vi "Automatic CE-CERT Inverter MODBUS TCP-IP Curtailment.vi"() -> ()   [LabVIEW 2018]
uses:
  <vilib>/Plasmionique/MB Master/MB_Master_TCP/MB_Master_TCP.lvclass
  C:/Program Files (x86)/National Instruments/LabVIEW 2018/vi.lib/Plasmionique/MB Master/MB_Master/MB_Master.lvclass
  <vilib>/Plasmionique/MB Master/MB Master.lvlib
panel:
  in  "Curtailment Percentage (28-100%)":u16
  out "3035 Register Value":u16
  out "Curtailment Mode Read Back (Step 11)":u16
  out "Power Factor Mode Read Back (Step 10)":u16
  out "Power Factor Operation Error (Step 9)(Can Read 0 or 10)":u16
  out "Power Factor Operation Error (Step 1)(Should Read 0)":u16
  in  "IP Address":string
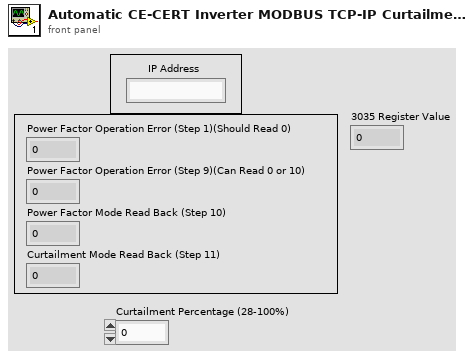
[diagram p1: front panel]
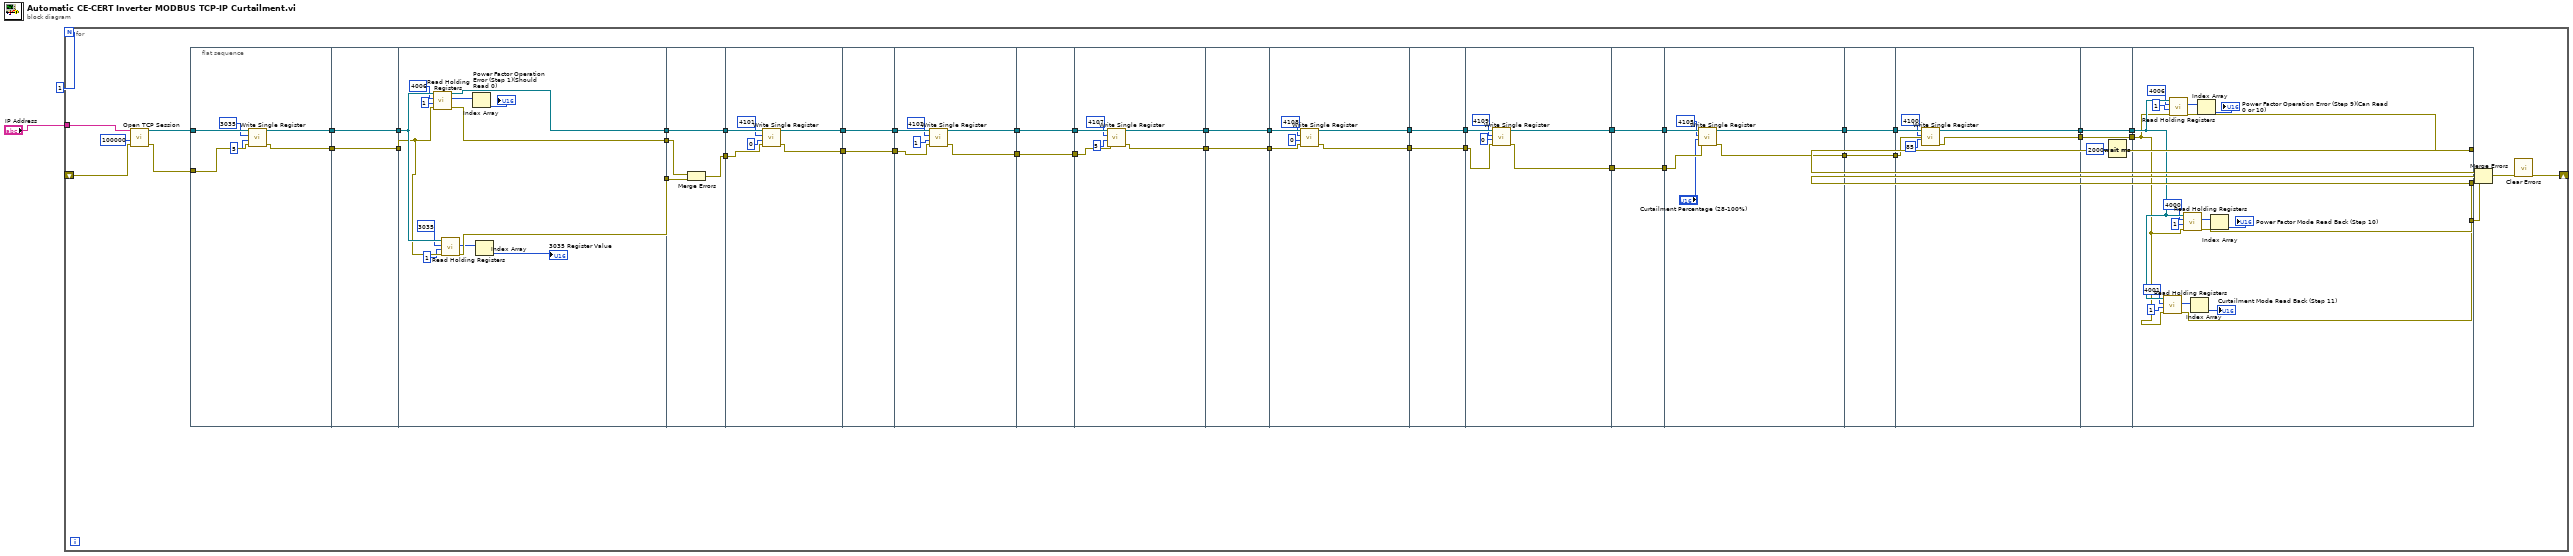
[diagram p0: block diagram]
diagram:
  n1 = for {
    N: 1 -> [_]
    tunnel: "IP Address" -> [w31]
    shift-right: [w5] -> _
    shift-left: _ -> [w4]
    n2 = call <vilib>:"Open TCP Session.vi"("error in (no error)"=w4, "Timeout (10000)"=100000, "IP Address"=w31) -> ("error out"=w29:errorcluster, "MB_TCP session"=w30:refnum<class "MB_Master_TCP.lvclass">)  [unwired: 7 in]
    n3 = flat-sequence {
      tunnel: w30 -> [w55]
      tunnel: [w54] -> w32
      tunnel: w29 -> [w53]
      tunnel: [w52] -> w27
      tunnel: [w57] -> w33
      tunnel: w32 -> [w57]
      tunnel: [w56] -> w28
      tunnel: w27 -> [w56]
      tunnel: [w70] -> w49
      tunnel: w33 -> [w69]
      tunnel: w28 -> [w68]
      tunnel: [w67] -> w25
      tunnel: [w66] -> w24
      tunnel: w49 -> [w74]
      tunnel: [w74] -> w48
      tunnel: [w71] -> w26
      tunnel: w25 -> [w73]
      tunnel: w24 -> [w72]
      tunnel: w48 -> [w80]
      tunnel: [w79] -> w47
      tunnel: w26 -> [w78]
      tunnel: [w77] -> w22
      tunnel: w47 -> [w82]
      tunnel: [w82] -> w46
      tunnel: [w81] -> w23
      tunnel: w22 -> [w81]
      tunnel: w46 -> [w88]
      tunnel: [w87] -> w45
      tunnel: w23 -> [w86]
      tunnel: [w85] -> w20
      tunnel: w45 -> [w90]
      tunnel: [w90] -> w44
      tunnel: [w89] -> w21
      tunnel: w20 -> [w89]
      tunnel: w44 -> [w96]
      tunnel: [w95] -> w43
      tunnel: w21 -> [w94]
      tunnel: [w93] -> w18
      tunnel: w43 -> [w98]
      tunnel: [w98] -> w42
      tunnel: [w97] -> w19
      tunnel: w18 -> [w97]
      tunnel: w42 -> [w104]
      tunnel: [w103] -> w41
      tunnel: w19 -> [w102]
      tunnel: [w101] -> w16
      tunnel: w41 -> [w106]
      tunnel: [w106] -> w40
      tunnel: [w105] -> w17
      tunnel: w16 -> [w105]
      tunnel: w40 -> [w112]
      tunnel: [w111] -> w39
      tunnel: w17 -> [w110]
      tunnel: [w109] -> w14
      tunnel: w39 -> [w114]
      tunnel: [w114] -> w38
      tunnel: [w113] -> w15
      tunnel: w14 -> [w113]
      tunnel: w38 -> [w120]
      tunnel: [w119] -> w37
      tunnel: w15 -> [w118]
      tunnel: [w117] -> w12
      tunnel: w37 -> [w122]
      tunnel: [w122] -> w36
      tunnel: [w121] -> w13
      tunnel: w12 -> [w121]
      tunnel: w36 -> [w128]
      tunnel: [w127] -> w35
      tunnel: w13 -> [w126]
      tunnel: [w125] -> w10
      tunnel: w35 -> [w131]
      tunnel: [w131] -> w34
      tunnel: [w129] -> w11
      tunnel: w10 -> [w129]
      tunnel: w34 -> [w148]
      tunnel: w11 -> [w147]
      tunnel: [w146] -> w8
      tunnel: [w145] -> w7
      tunnel: [w144] -> w6
      frame #0 {
        n4 = call <vilib>:"Write Single Register.vi"("error in (no error)"=w53, "value"=u16 5, "address"=u16 3035, "MB session in"=w55) -> ("error out"=w52:errorcluster, "MB session out"=w54:refnum<class "MB_Master_TCP.lvclass">)  [unwired: 6 in]
      }
      frame #1 {
      }
      frame #2 {
        n5 = call <vilib>:"Read Holding Registers.vi"("error in (no error)"=w68, "quantity"=u16 1, "starting address"=u16 4006, "MB session in"=w69) -> ("error out"=w67:errorcluster, "Registers"=w61:u16[], "MB session out"=w70:refnum<class "MB_Master_TCP.lvclass">)  [unwired: 5 in]
        n6 = call <vilib>:"Read Holding Registers.vi"("error in (no error)"=w68, "quantity"=u16 1, "starting address"=u16 3035, "MB session in"=w69) -> ("error out"=w66:errorcluster, "Registers"=w63:u16[])  [unwired: 5 in, 1 out]
        n7 = Index Array(array=w61) -> (element=→"Power Factor Operation Error (Step 1)(Should Read 0)":u16)  [unwired: 1 in]
        n8 = Index Array(array=w63) -> (element=→"3035 Register Value":u16)  [unwired: 1 in]
      }
      frame #3 {
        n9 = Merge Errors(w73, w72) -> (w71:errorcluster)
      }
      frame #4 {
        n10 = call <vilib>:"Write Single Register.vi"("error in (no error)"=w78, "value"=u16 0, "address"=u16 4101, "MB session in"=w80) -> ("error out"=w77:errorcluster, "MB session out"=w79:refnum<class "MB_Master_TCP.lvclass">)  [unwired: 6 in]
      }
      frame #5 {
      }
      frame #6 {
        n11 = call <vilib>:"Write Single Register.vi"("error in (no error)"=w86, "value"=u16 1, "address"=u16 4102, "MB session in"=w88) -> ("error out"=w85:errorcluster, "MB session out"=w87:refnum<class "MB_Master_TCP.lvclass">)  [unwired: 6 in]
      }
      frame #7 {
      }
      frame #8 {
        n12 = call <vilib>:"Write Single Register.vi"("error in (no error)"=w94, "value"=u16 5, "address"=u16 4107, "MB session in"=w96) -> ("error out"=w93:errorcluster, "MB session out"=w95:refnum<class "MB_Master_TCP.lvclass">)  [unwired: 6 in]
      }
      frame #9 {
      }
      frame #10 {
        n13 = call <vilib>:"Write Single Register.vi"("error in (no error)"=w102, "value"=u16 0, "address"=u16 4108, "MB session in"=w104) -> ("error out"=w101:errorcluster, "MB session out"=w103:refnum<class "MB_Master_TCP.lvclass">)  [unwired: 6 in]
      }
      frame #11 {
      }
      frame #12 {
        n14 = call <vilib>:"Write Single Register.vi"("error in (no error)"=w110, "value"=u16 0, "address"=u16 4109, "MB session in"=w112) -> ("error out"=w109:errorcluster, "MB session out"=w111:refnum<class "MB_Master_TCP.lvclass">)  [unwired: 6 in]
      }
      frame #13 {
      }
      frame #14 {
        n15 = call <vilib>:"Write Single Register.vi"("error in (no error)"=w118, "value"="Curtailment Percentage (28-100%)", "address"=u16 4105, "MB session in"=w120) -> ("error out"=w117:errorcluster, "MB session out"=w119:refnum<class "MB_Master_TCP.lvclass">)  [unwired: 6 in]
      }
      frame #15 {
      }
      frame #16 {
        n16 = call <vilib>:"Write Single Register.vi"("error in (no error)"=w126, "value"=u16 85, "address"=u16 4100, "MB session in"=w128) -> ("error out"=w125:errorcluster, "MB session out"=w127:refnum<class "MB_Master_TCP.lvclass">)  [unwired: 6 in]
      }
      frame #17 {
        n17 = Wait (ms)(milliseconds to wait=u32 2000) -> ()  [unwired: 1 out]
      }
      frame #18 {
        n18 = call <vilib>:"Read Holding Registers.vi"("error in (no error)"=w147, "quantity"=u16 1, "starting address"=u16 4001, "MB session in"=w148) -> ("error out"=w144:errorcluster, "Registers"=w133:u16[])  [unwired: 5 in, 1 out]
        n19 = call <vilib>:"Read Holding Registers.vi"("error in (no error)"=w147, "quantity"=u16 1, "starting address"=u16 4006, "MB session in"=w148) -> ("error out"=w146:errorcluster, "Registers"=w141:u16[])  [unwired: 5 in, 1 out]
        n20 = call <vilib>:"Read Holding Registers.vi"("error in (no error)"=w147, "quantity"=u16 1, "starting address"=u16 4000, "MB session in"=w148) -> ("error out"=w145:errorcluster, "Registers"=w137:u16[])  [unwired: 5 in, 1 out]
        n21 = Index Array(array=w133) -> (element=→"Curtailment Mode Read Back (Step 11)":u16)  [unwired: 1 in]
        n22 = Index Array(array=w141) -> (element=→"Power Factor Operation Error (Step 9)(Can Read 0 or 10)":u16)  [unwired: 1 in]
        n23 = Index Array(array=w137) -> (element=→"Power Factor Mode Read Back (Step 10)":u16)  [unwired: 1 in]
      }
    }
    n24 = Merge Errors(w8, w7, w6) -> (w9:errorcluster)
    n25 = call <vilib>:"Clear Errors.vi"("error in (no error)"=w9) -> ("error out"=w5:errorcluster)  [unwired: 5 in, 1 out]
  }
